vi "inst.Optos.vi"(8 "error in (no error)":errorcluster, 11 "Modbus master in":refnum<class "Modbus Master.lvclass">) -> (0 "error out":errorcluster, 1 "inputs":bool[](array[boolean]), 2 "short circuits":bool[](array[boolean]), 3 "Modbus master out":refnum<class "Modbus Master.lvclass">)   [LabVIEW 2018, in "MB Relay.lvlib"]
uses:
  MB Relay.lvlib
  <vilib>/NI/Modbus Library/API/Master/Modbus Master.lvclass
  type defs/MB relays _InstrumentType.ctl
  type defs/FGV enum.ctl
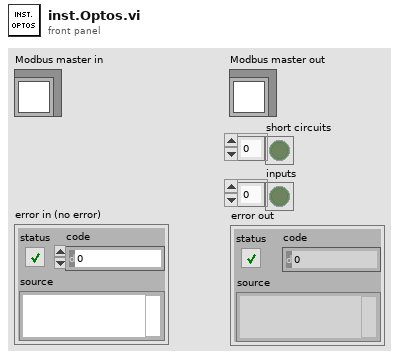
[diagram p1: front panel]
types:
  T1 = typedef "MB Relay.lvlib/FGV enum.ctl" = enum16{"Write", "Read", "All OFF", "All ON"}
  T2 = typedef "MB Relay.lvlib/MB relays _InstrumentType.ctl" = enum16{"counter", "demux1_10(x6)", "mux10_1(x6)", "mux6_1(3wires)", "MB_Relay_01", "SpareRelays", "Optos", "Inputs", "DMM I 0.5", "5V enable"}
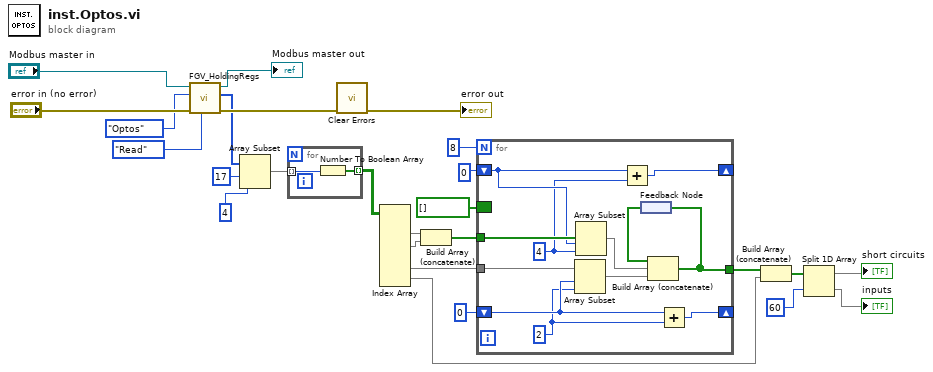
[diagram p0: block diagram]
diagram:
  n1 = call "FGV_HoldingRegs.vi"("FGV_enum"=FGV_enum."Read", "error in (no error)"="error in (no error)", "Instruments"=MB_relays__InstrumentType."Optos", "Modbus master in"="Modbus master in") -> ("error out"=w11:errorcluster, "HoldingRegs"=w7:u16[], "Modbus master out"=→"Modbus master out":refnum<class "Modbus Master.lvclass">)  [unwired: 5 in]
  n2 = Array Subset(array=w7, index=17, length=4) -> (w4:u16[])
  n3 = for {
    tunnel: [w28] -> w24 mode=indexing
    tunnel: w4 -> [w27] mode=indexing
    n4 = Number To Boolean Array(number=w27) -> (Boolean array=w28:bool[])
  }
  n5 = call <vilib>:"Clear Errors.vi"("error in (no error)"=w11) -> ("error out"=→"error out":errorcluster)  [unwired: 5 in, 1 out]
  n6 = Index Array(array=w24) -> (element #1=w22:bool[], element #2=w23:bool[], element #3=w19:bool[], element #4=w18:bool[])  [unwired: 8 in]
  n7 = Build Array (concatenate)(w22, w23) -> (w21:bool[])
  n8 = for {
    N: 8 -> [_]
    tunnel: w21 -> [w40]
    tunnel: w19 -> [w36]
    shift-right: [w37] -> _
    shift-left: 0 ("length") -> [w39]
    shift-right: [w33] -> _
    shift-left: 0 ("length") -> [w35]
    tunnel: [w29] -> w14
    border: bool[] [] -> [_]
    w34 = 2 ("length")
    w38 = 4 ("length")
    n9 = Array Subset(array=w36, index=w35, length=w34) -> (w32:bool[])
    n10 = Array Subset(array=w40, index=w39, length=w38) -> (w31:bool[])
    n11 = Add(x=w39, y=w38) -> (x+y=w37:i32)
    n12 = feedback #1() -> (w30:bool[])
    n13 = Build Array (concatenate)(w30, w31, w32) -> (w29:bool[])
    n14 = feedback-in #1(w29) -> ()
    n15 = Add(x=w35, y=w34) -> (x+y=w33:i32)
  }
  n16 = Build Array (concatenate)(w14, w18) -> (w10:bool[])
  n17 = Split 1D Array(array=w10, index=60) -> (first subarray=→"short circuits":bool[], second subarray=→"inputs":bool[])
